vi "Update Scenarios Table for Spartan 5.0.vi"(8 "error in (no error)":errorcluster, 11 "Connection Refnum":T1) -> (0 "error out":errorcluster, 3 "Connection Refnum":T1)   [LabVIEW 2011]
uses:
  Summitek EXT/ODBC/SQL Controls/Connection Refnum.ctl
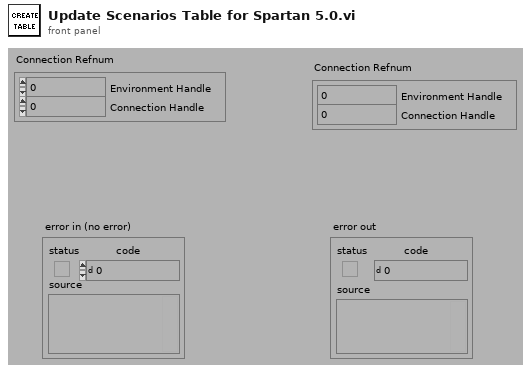
[diagram p1: front panel]
types:
  T1 = typedef "Connection Refnum.ctl" = cluster{"Environment Handle":i32, "Connection Handle":i32}
  T2 = typedef "Statement Refnum.ctl" = cluster{"Statement Handle":i32, "Parameter Number":u16}
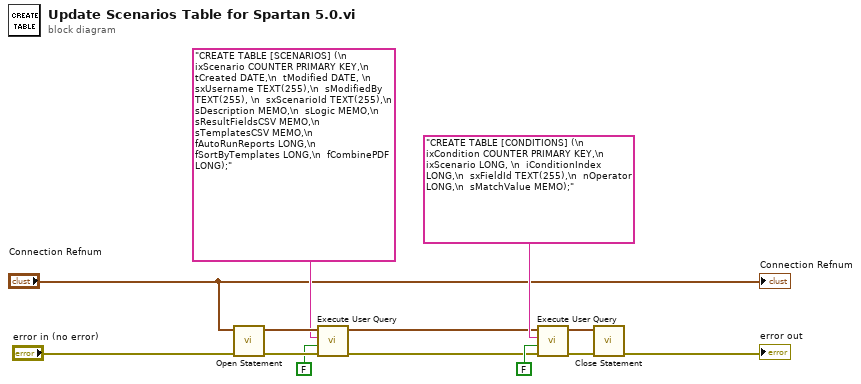
[diagram p0: block diagram]
diagram:
  n1 = call "Open Statement.vi"("error in (no error)"="error in (no error)", "Connection Refnum"="Connection Refnum") -> ("error out"=w13:errorcluster, "Statement Refnum"=w12:T2)  [unwired: 4 out]
  n2 = call "Execute User Query.vi"("error in (no error)"=w13, "Return Data? (f)"=FALSE, "User Query"="CREATE TABLE [SCENARIOS] (\n  ixScenario COUNTER PRIMARY KEY,\n  tCreated DATE,\n  tModified DATE, \n  sxUsername TEXT(255),\n  sModifiedBy TEXT(255), \n  sxScenarioId TEXT(255),\n  sDescription MEMO,\n  sLogic MEMO,\n  sResultFieldsCSV MEMO,\n  sTemplatesCSV MEMO,\n  fAutoRunReports LONG,\n  fSortByTemplates LONG,\n  fCombinePDF LONG);", "Statement Refnum"=w12) -> ("error out"=w1:errorcluster, "Statement Refnum"=w2:T2)  [unwired: 2 out]
  n3 = call "Execute User Query.vi"("error in (no error)"=w1, "Return Data? (f)"=FALSE, "User Query"="CREATE TABLE [CONDITIONS] (\n  ixCondition COUNTER PRIMARY KEY,\n  ixScenario LONG, \n  iConditionIndex LONG,\n  sxFieldId TEXT(255),\n  nOperator LONG,\n  sMatchValue MEMO);", "Statement Refnum"=w2) -> ("error out"=w7:errorcluster, "Statement Refnum"=w8:T2)  [unwired: 2 out]
  n4 = call "Close Statement.vi"("error in (no error)"=w7, "Statement Refnum"=w8) -> ("error out"=→"error out":errorcluster)  [unwired: 5 out]
  "Connection Refnum" <- "Connection Refnum"
